vi "Result Handling FGV.vi"(8 "error in":errorcluster, 10 "Test Result In":T1={"Test Frequency"=12750, "Received Packets"=0, "Results"="", "Test Paramaters"={"Interference sig. freq."=30, "Wanted Signal"=-67.0, "Blocking Signal"=-67.0, "Measurement res."=10}} {"Test Paramaters"."Measurement res." format="%.0f MHz"; "Test Paramaters"."Blocking Signal" format="%#_gdBm"; "Test Paramaters"."Interference sig. freq." format="%.0f MHz"; "Test Paramaters"."Wanted Signal" format="%#_gdBm"; "Test Frequency" format="%.0f MHz"}, 11 "Command":T3) -> (0 "error out":errorcluster, 2 "Result Array":T1[](array[typedef]) {"Test Paramaters"."Measurement res." format="%.0f MHz"; "Test Paramaters"."Blocking Signal" format="%#_gdBm"; "Test Paramaters"."Interference sig. freq." format="%.0f MHz"; "Test Paramaters"."Wanted Signal" format="%#_gdBm"; "Test Frequency" format="%.0f MHz"})   [LabVIEW 2013]
doc: "This Fuctional Global Variable will record results and return certain sets fo the data."
uses:
  Results FGV Command.ctl
  Test Results Cluster.ctl
  Test Parameters.ctl
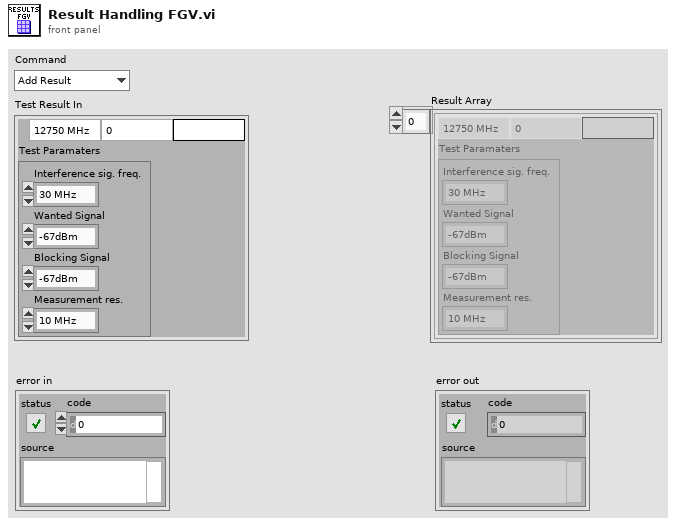
[diagram p1: front panel]
types:
  T1 = typedef "Test Results Cluster.ctl" = cluster{"Test Frequency":u32, "Received Packets":u32, "Results":string, "Test Paramaters":T2}
  T2 = typedef "Test Parameters.ctl" = cluster{"Interference sig. freq.":u32, "Wanted Signal":dbl, "Blocking Signal":dbl, "Measurement res.":u32}
  T3 = typedef "Results FGV Command.ctl" = enum16{"Add Result", "Return All", "Return fbf_1", "Return fbf_2", "Replace", "Clear All"}
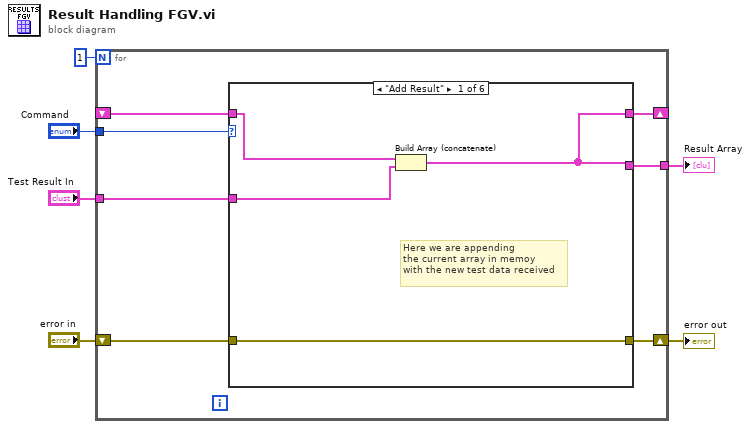
[diagram p0: block diagram]
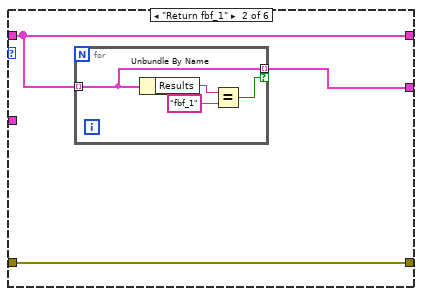
[diagram p2: hidden frame]
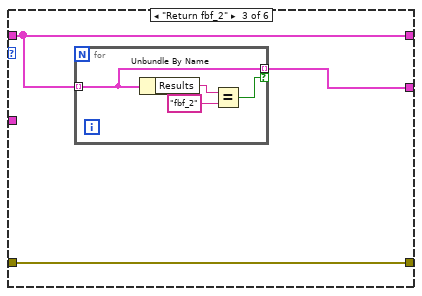
[diagram p3: hidden frame]
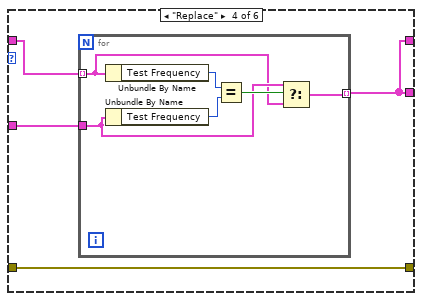
[diagram p4: hidden frame]
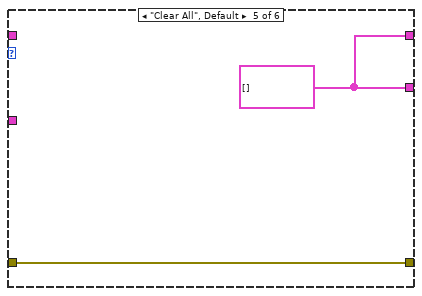
[diagram p5: hidden frame]
diagram:
  n1 = for {
    N: 1 -> [_]
    tunnel: "Command" -> [w13]
    tunnel: "Test Result In" -> [w11]
    shift-right: [w10] -> _
    shift-left: _ -> [w7]
    tunnel: [w9] -> w2
    shift-right: [w12] -> w5
    shift-left: "error in" -> [w8]
    n2 = case shown="\"Add Result\"" w13 {
      tunnel: w8 -> [w17 w18 w25 w32 w43 w44]
      tunnel: [w17 w18 w25 w32 w43 w44] -> w12
      tunnel: w11 -> [w15 _ _ w34 _ _]
      tunnel: [w14 w19 w26 w33 w42 w45] -> w10
      tunnel: [w14 w20 w27 w33 w42 w45] -> w9
      tunnel: w7 -> [w16 w19 w26 w35 _ w45]
      frame "Add Result" {
        # "Here we are appending\nthe current array in memoy\nwith the new test data received"
        n3 = Build Array (concatenate)(w16, w15) -> (w14:T1[])
      }
      frame "Return fbf_1" {
        n4 = for {
          tunnel: w19 -> [w22] mode=indexing
          tunnel: [w22] -> w20 mode=indexing if=w21
          n5 = Unbundle By Name(w22) -> ("Results"=w24:string)
          n6 = Equal?(x=w24, y="fbf_1") -> (x = y?=w21:bool)
        }
      }
      frame "Return fbf_2" {
        n7 = for {
          tunnel: w26 -> [w29] mode=indexing
          tunnel: [w29] -> w27 mode=indexing if=w28
          n8 = Unbundle By Name(w29) -> ("Results"=w31:string)
          n9 = Equal?(x=w31, y="fbf_2") -> (x = y?=w28:bool)
        }
      }
      frame "Replace" {
        n10 = for {
          tunnel: w35 -> [w37] mode=indexing
          tunnel: w34 -> [w38]
          tunnel: [w36] -> w33 mode=indexing
          n11 = Unbundle By Name(w37) -> ("Test Frequency"=w41:u32)
          n12 = Unbundle By Name(w38) -> ("Test Frequency"=w40:u32)
          n13 = Equal?(x=w41, y=w40) -> (x = y?=w39:bool)
          n14 = Select(t=w38, s=w39, f=w37) -> (s? t:f=w36:T1)
        }
      }
      frame "Clear All", Default {
        w42 = T1[] [] ("Result Array")
      }
      frame "Return All" {
      }
    }
  }
  "error out" <- w5
  "Result Array" <- w2
